vi "InitialiseDevice.vi"(8 "error In":errorcluster, 9 "PicoMotor IP In":string) -> (0 "error out":errorcluster, 1 "DreviceAddressOut":i32, 2 "DeviceKey Out":string, 3 "CmdLib Out":refnum<k24>)   [LabVIEW 2020]
uses:
  C:/GEECS/Developers Version/builds/Device builds/Picomotor8742dotNet/CmdLib.dll
  CmdLib.dll
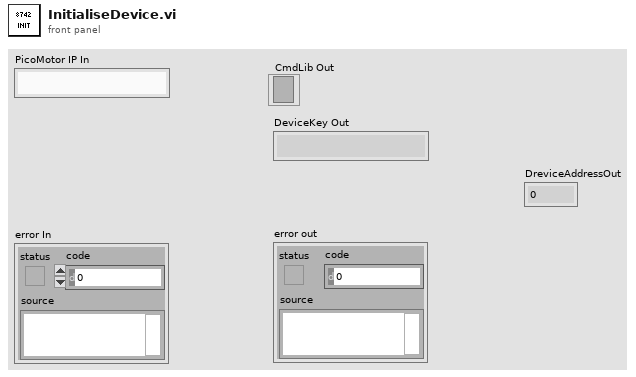
[diagram p1: front panel]
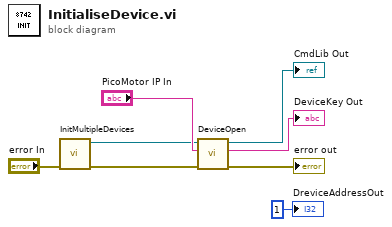
[diagram p0: block diagram]
diagram:
  n1 = call "InitMultipleDevices.vi"("error in (no error)"="error In") -> ("error out"=w3:errorcluster, "CmdLib Out"=w4:refnum<k24>)  [unwired: 5 in]
  n2 = call "DeviceOpen.vi"("error in (no error)"=w3, "DeviceKey In"="PicoMotor IP In", "CmdLib In"=w4) -> ("error out"=→"error out":errorcluster, "DeviceKey Out"=→"DeviceKey Out":string, "CmdLib Out"=→"CmdLib Out":refnum<k24>)  [unwired: 2 in]
  "DreviceAddressOut" <- 1 ("DreviceAddressOut")
